vi "Create.vi"(10 "MultiErrors":refnum<class "MultiErrors.lvclass">) -> (3 "MultiError Value out":refnum<class "MultiError Value.lvclass">)   [LabVIEW 2020, in "Volatus.lvlib" / "MultiError Value.lvclass"]
uses:
  MultiError Value.lvclass
  MultiError Value.lvclass/MultiError Value.ctl
  MultiErrors/MultiErrors.lvclass
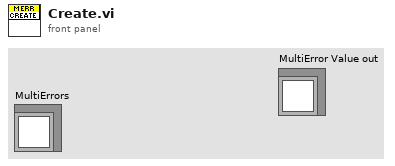
[diagram p1: front panel]
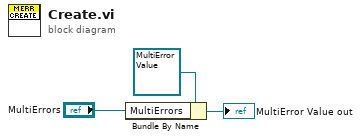
[diagram p0: block diagram]
diagram:
  n1 = Bundle By Name(cluster=refnum<class "MultiError Value.lvclass"> refnum ("MultiError Value in"), "MultiErrors"="MultiErrors") -> (→"MultiError Value out":refnum<class "MultiError Value.lvclass">)
